vi "main.vi"(8 "error in (no error)":errorcluster, 9 "Power":sgl=100.0, 10 "PRR":sgl, 11 "Laser_Ethernet in":refnum<class "Laser_Ethernet.lvclass">) -> (0 "error out":errorcluster, 3 "Laser_Ethernet out":refnum<class "Laser_Ethernet.lvclass">)   [LabVIEW 2023, in "Laser_Ethernet.lvclass"]
uses:
  Laser_Ethernet.lvclass
  Laser_Ethernet.lvclass/Laser_Ethernet.ctl
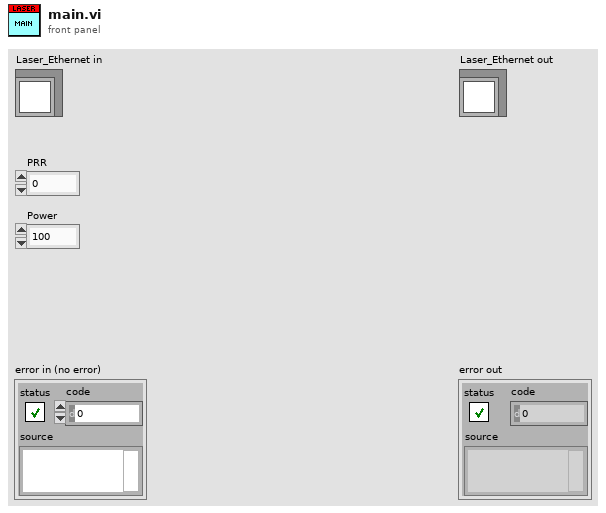
[diagram p1: front panel]
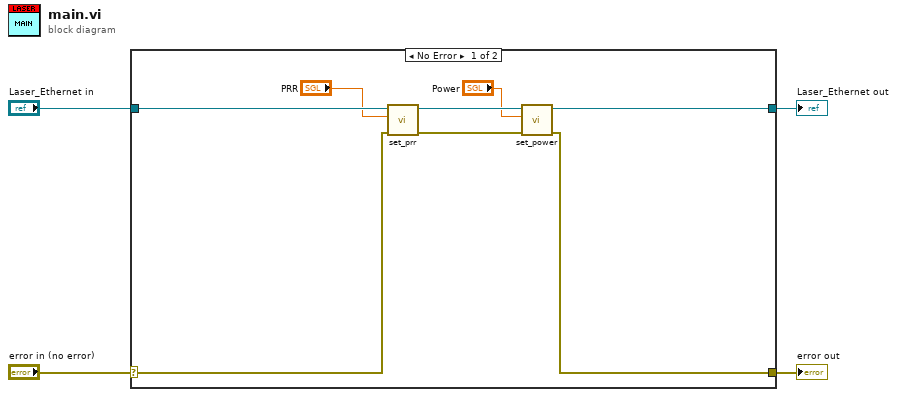
[diagram p0: block diagram]
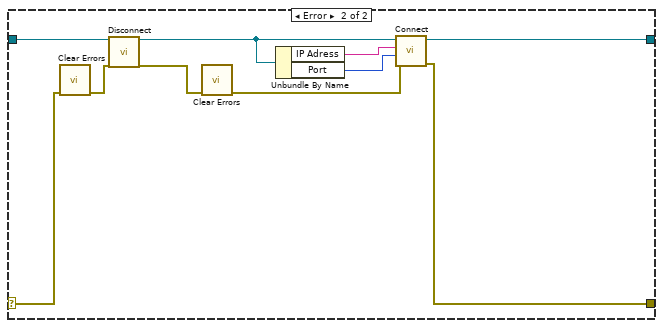
[diagram p2: hidden frame]
diagram:
  n1 = case shown="No Error" "error in (no error)" {
    selector: "error in (no error)" -> [w11 w21]
    tunnel: [w6 w14] -> w3
    tunnel: [w8 w13] -> w1
    tunnel: "Laser_Ethernet in" -> [w12 w22]
    frame No Error {
      n2 = call-dynamic "set_prr.vi"("error in (no error)"=w11, "PRR"="PRR", "Laser_Ethernet in"=w12) -> ("error out"=w7:errorcluster, "Laser_Ethernet out"=w9:refnum<class "Laser_Ethernet.lvclass">)  [unwired: 7 in]
      n3 = call-dynamic "set_power.vi"("error in (no error)"=w7, "Power"="Power", "Laser_Ethernet in"=w9) -> ("error out"=w6:errorcluster, "Laser_Ethernet out"=w8:refnum<class "Laser_Ethernet.lvclass">)  [unwired: 7 in]
    }
    frame Error {
      n4 = call <vilib>:"Clear Errors.vi"("error in (no error)"=w21) -> ("error out"=w20:errorcluster)  [unwired: 5 in, 1 out]
      n5 = call-dynamic "Disconnect.vi"("object in"=w22, "error in (no error)"=w20) -> ("object out"=w17:refnum<class "Laser_Ethernet.lvclass">, "error out"=w19:errorcluster)  [unwired: 16 in]
      n6 = call <vilib>:"Clear Errors.vi"("error in (no error)"=w19) -> ("error out"=w18:errorcluster)  [unwired: 5 in, 1 out]
      n7 = Unbundle By Name(w17) -> ("IP Adress"=w16:string, "Port"=w15:u16)
      n8 = call-dynamic "Connect.vi"("error in (no error)"=w18, "remote port or service name"=w15, "address"=w16, "object in"=w17) -> ("error out"=w14:errorcluster, "object out"=w13:refnum<class "Laser_Ethernet.lvclass">)  [unwired: 5 in, 1 out]
    }
  }
  "error out" <- w3
  "Laser_Ethernet out" <- w1
